vi "Mapping Error Handler (Single).vi"(8 "error in (no error)":errorcluster, 11 "Mapping Error":T1) -> (0 "error out":errorcluster, 3 "Continue?":bool)   [LabVIEW 2016, in "System Mapping Tool.lvlib"]
uses:
  System Mapping Tool.lvlib
  TypeDefs/Mapping Error Cluster.ctl
  TypeDefs/Mapping Error.ctl
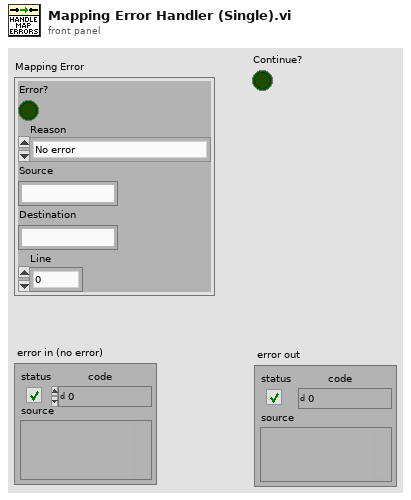
[diagram p1: front panel]
types:
  T1 = typedef "System Mapping Tool.lvlib/Mapping Error Cluster.ctl" = cluster{"Error?":bool, "Reason":T2, "Source":string, "Destination":string, "Line":i32}
  T2 = typedef "System Mapping Tool.lvlib/Mapping Error.ctl" = enum16{"No error", "Channels already mapped", "Source is not valid", "Destination is not valid", "Destination already mapped", "Destination mapped twice"}
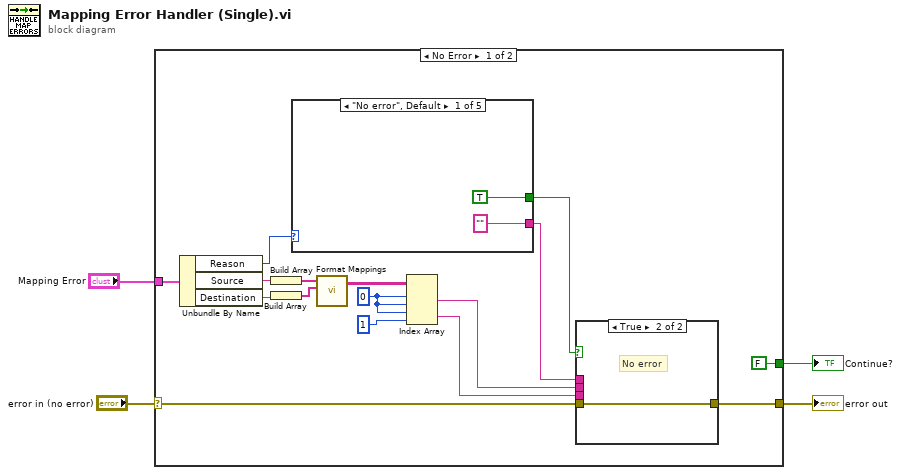
[diagram p0: block diagram]
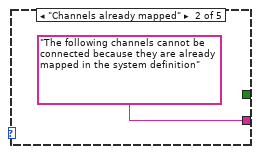
[diagram p2: hidden frame]
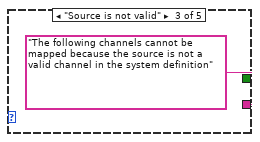
[diagram p3: hidden frame]
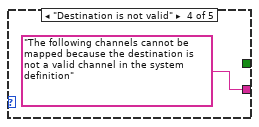
[diagram p4: hidden frame]
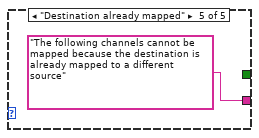
[diagram p5: hidden frame]
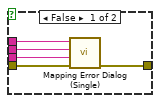
[diagram p6: hidden frame]
diagram:
  n1 = case shown="No Error" "error in (no error)" {
    selector: "error in (no error)" -> [w12 w33]
    tunnel: [w13 w33] -> w3
    tunnel: "Mapping Error" -> [w20 _]
    tunnel: [FALSE ("Continue?") _] -> w2
    frame No Error {
      w9 = 0 ("index (row)")
      n2 = Unbundle By Name(w20) -> ("Reason"=w19:T2, "Source"=w18:string, "Destination"=w16:string)
      n3 = Build Array(w18) -> (w17:string[])
      n4 = Build Array(w16) -> (w15:string[])
      n5 = case shown="\"No error\", Default" w19 {
        tunnel: ["" "The following channels cannot be connected because they are already mapped in the system definition" "The following channels cannot be mapped because the source is not a valid channel in the system definition" "The following channels cannot be mapped because the destination is not a valid channel in the system definition" "The following channels cannot be mapped because the destination is already mapped to a different source"] -> w11
        tunnel: [TRUE _ _ _ _] -> w5
        frame "No error", Default {
        }
        frame "Channels already mapped" {
        }
        frame "Source is not valid" {
        }
        frame "Destination is not valid" {
        }
        frame "Destination already mapped" {
        }
      }
      n6 = call "Format Mappings.vi"("Destinations"=w15, "Sources"=w17) -> ("Mappings"=w14:string[][])  [unwired: 3 in]
      n7 = Index Array(array=w14, index (row) #1=w9, index (col) #1=w9, index (row) #2=w9, index (col) #2=1 ("index (row)")) -> (element #1=w8:string, element #2=w7:string)
      n8 = case shown="True" w5 {
        tunnel: [w31 w32] -> w13
        tunnel: w12 -> [w30 w32]
        tunnel: w11 -> [w29 _]
        tunnel: w8 -> [w28 _]
        tunnel: w7 -> [w27 _]
        frame False {
          n9 = call "Mapping Error Dialog (Single).vi"("error in (no error)"=w30, "Destination"=w27, "Source"=w28, "Error Text"=w29) -> ("error out"=w31:errorcluster)  [unwired: 7 in]
        }
        frame True {
          # "No error"
        }
      }
    }
    frame Error {
    }
  }
  "error out" <- w3
  "Continue?" <- w2
